vi "get_timestamp.vi"() -> (1 "unix time (seconds since the epoch)":u32, 2 "time string":string, 3 "date string":string)   [LabVIEW 2018]
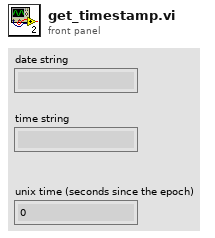
[diagram p1: front panel]
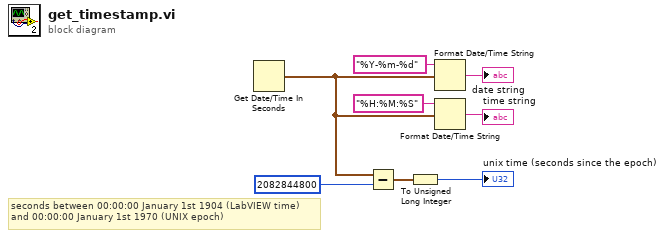
[diagram p0: block diagram]
diagram:
  # "seconds between 00:00:00 January 1st 1904 (LabVIEW time)\nand 00:00:00 January 1st 1970 (UNIX epoch)"
  n1 = Get Date/Time In Seconds() -> (seconds since 1Jan1904=w2:timestamp)
  n2 = Subtract(x=w2, y=u32 2082844800) -> (x-y=w5:timestamp)
  n3 = To Unsigned Long Integer(number=w5) -> (unsigned 32bit integer=→"unix time (seconds since the epoch)":u32)
  n4 = Format Date/Time String(time format string (%c)="%Y-%m-%d", seconds (now)=w2) -> (date/time string=→"date string":string)  [unwired: 1 in]
  n5 = Format Date/Time String(time format string (%c)="%H:%M:%S", seconds (now)=w2) -> (date/time string=→"time string":string)  [unwired: 1 in]
